vi "tm3samp_snap_electron.vi"() -> ()   [LabVIEW 2012]
panel:
  out "Offset":sgl
  out "Coefficient":sgl
  out "Image":sgl[][](graph)
  out "Error Out":errorcluster
  # "This example shows how to\ntake a snapped image and\nconvert the data to electrons.\nElectron conversion data is not\navailable for all cameras."
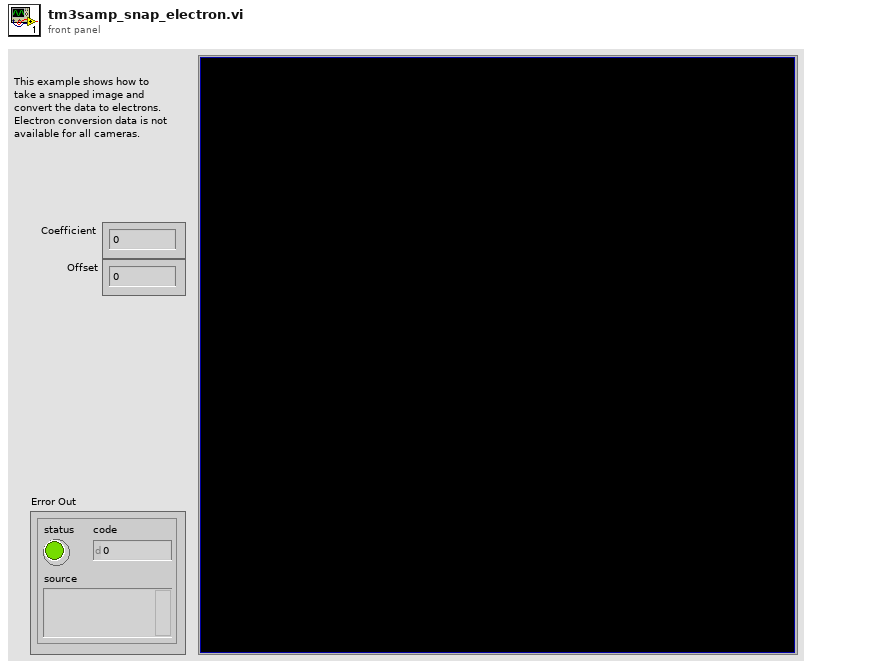
[diagram p1: front panel]
types:
  T1 = cluster{"width":u32, "height":u32, "datatype":u32}
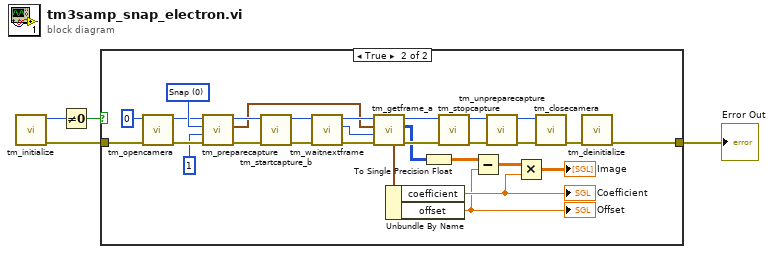
[diagram p0: block diagram]
diagram:
  n1 = call <userlib>:"tm_initialize.vi"() -> ("error out"=w1:errorcluster, "Number Of Cameras"=w2:u32)  [unwired: 10 in]
  n2 = Not Equal To 0?(x=w2) -> (x != 0?=w4:bool)
  n3 = case shown="True" w4 {
    tunnel: w1 -> [w5 w34]
    tunnel: [w5 w31] -> w3
    frame False {
    }
    frame True {
      w26 = 0 items=["Snap", "Sequence"] ("Capture mode")
      n4 = call <userlib>:"tm_opencamera.vi"("error in (no error)"=w34, "Camera Index"=u32 0) -> ("error out"=w22:errorcluster, "Handle out"=w23:u32)  [unwired: 8 in]
      n5 = call <userlib>:"tm_preparecapture.vi"("error in (no error)"=w22, "Frames"=1, "Capture mode"=w26, "Handle in"=w23) -> ("error out"=w24:errorcluster, "Buffer"=w16:T1, "Handle out"=w25:u32)  [unwired: 4 in, 1 out]
      n6 = call <userlib>:"tm_startcapture_b.vi"("error in (no error)"=w24, "Handle in"=w25) -> ("error out"=w20:errorcluster, "Handle out"=w19:u32)  [unwired: 8 in]
      n7 = call <userlib>:"tm_waitnextframe.vi"("error in (no error)"=w20, "Handle in"=w19) -> ("error out"=w18:errorcluster, "Frame Index"=w15:i32, "Handle out"=w17:u32)  [unwired: 6 in, 1 out]
      n8 = call <userlib>:"tm_getframe_a.vi"("error in (no error)"=w18, "Frame Index"=w15, "Buffer"=w16, "Handle in"=w17) -> ("error out"=w13:errorcluster, "Data 16"=w10:u16[][], "Handle out"=w14:u32, "Electron Info"=w11:cluster{"coefficient":sgl, "offset":sgl})  [unwired: 3 in, 1 out]
      n9 = Unbundle By Name(w11) -> ("coefficient"=w7:sgl, "offset"=w6:sgl)
      "Offset" <- w6
      "Coefficient" <- w7
      n10 = To Single Precision Float(number=w10) -> (single precision float=w9:sgl[][])
      n11 = call <userlib>:"tm_stopcapture.vi"("error in (no error)"=w13, "Handle in"=w14) -> ("error out"=w27:errorcluster, "Handle out"=w28:u32)  [unwired: 8 in]
      n12 = Subtract(x=w9, y=w6) -> (x-y=w12:sgl[][])
      n13 = call <userlib>:"tm_unpreparecapture.vi"("error in (no error)"=w27, "Handle in"=w28) -> ("error out"=w30:errorcluster, "Handle out"=w29:u32)  [unwired: 8 in]
      n14 = Multiply(x=w12, y=w7) -> (x*y=→"Image":sgl[][])
      n15 = call <userlib>:"tm_closecamera.vi"("error in (no error)"=w30, "Handle in"=w29) -> ("error out"=w32:errorcluster)  [unwired: 9 in]
      n16 = call <userlib>:"tm_deinitialize.vi"("error in (no error)"=w32) -> ("error out"=w31:errorcluster)  [unwired: 10 in]
    }
  }
  "Error Out" <- w3
